vi "LS Data Loop.vi"(11 "FPGA Ref":T1) -> ()   [LabVIEW 2013]
uses:
  Controls/FPGA_Reference.ctl
  <vilib>/rvi/interface/common/niFpgaWaitOnOcc.vi
  <vilib>/Utility/error.llb/Error Cluster From Error Code.vi
  <vilib>/rvi/errors/niLvFpgaAdjustHostInterfaceError.vi
  <vilib>/rvi/interface/nirviMethod/nirviMethod.xnode
  FPGA Bitfiles/LSDurability_Main.lvbitx
  <vilib>/rvi/interface/nirviReadWriteControl/nirviReadWriteControl.xnode
  <vilib>/FPGAPlugInAG/sbRIO-9626/niLvFpga_ReadFifo_sbRIO-9626.vi
  <vilib>/rvi/errors/niLvFpgaMergeErrorWithErrorCode.vi
  NiFpgaLv.dll
panel:
  in  "LoopWait(ms) 2":u32=100
  in  "Sections 2":i32=100
  out "FIFO loops 2":i32
  out "FIFO loops":i32
  in  "LoopWait(ms)":u32=100
  in  "Sections":i32=100
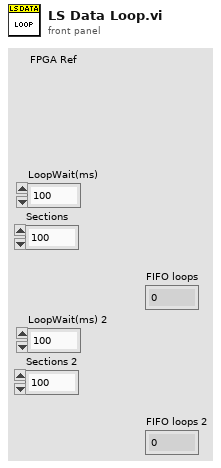
[diagram p1: front panel]
types:
  T1 = typedef "FPGA_Reference.ctl" = refnum<k20>
  T2 = cluster{"FPGA Ref":T1, "Time":dbl, "PtsTaken":i32, "Pts/File":i32, "10AveWait":u32, "Stored Filepath":path, "FileIndex":i32, "FilesUsed":i32, "Day":i32, "Anomaly Path":path}
  T3 = enum16{"open", "replace", "create", "open or create", "replace or create", "replace or create with confirmation"}
  T4 = cluster{"Running?":bool, "Profile Record":bool, "RecordInterval":i32, "RecordDuration":i32, "RecordFreq":i32, "Data Filepath":path, "Hr Record":bool, "Serial Numbers":string[]}
  T5 = typedef "LVDateTimeRec.ctl" = cluster{"fractional second":dbl, "second":i32, "minute":i32, "hour":i32, "day of month":i32, "month":i32, "year":i32, "day of week":i32, "day of year":i32, "DST":i32}
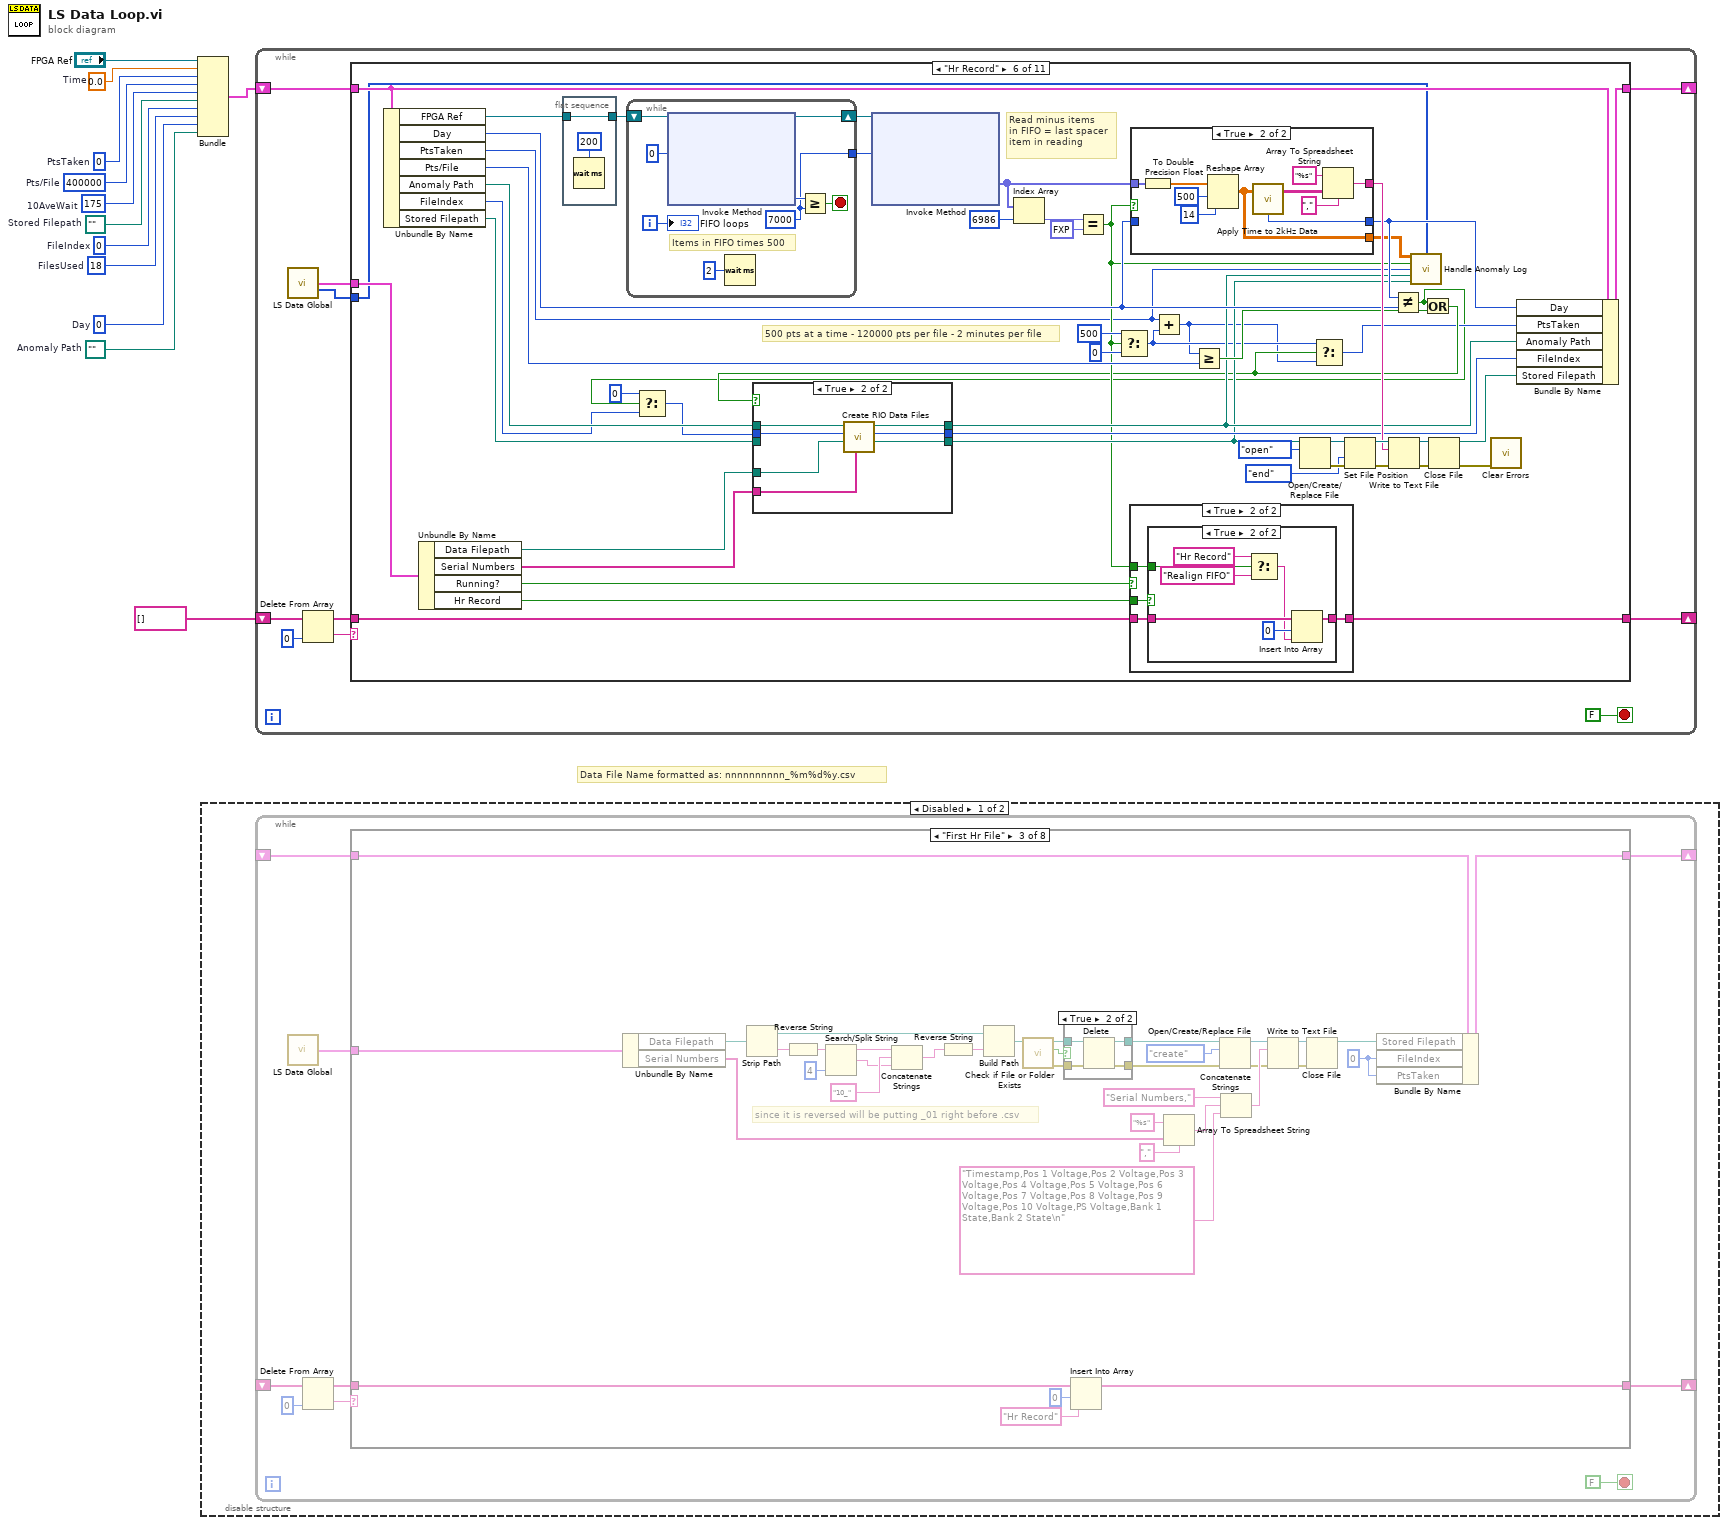
[diagram p0: block diagram]
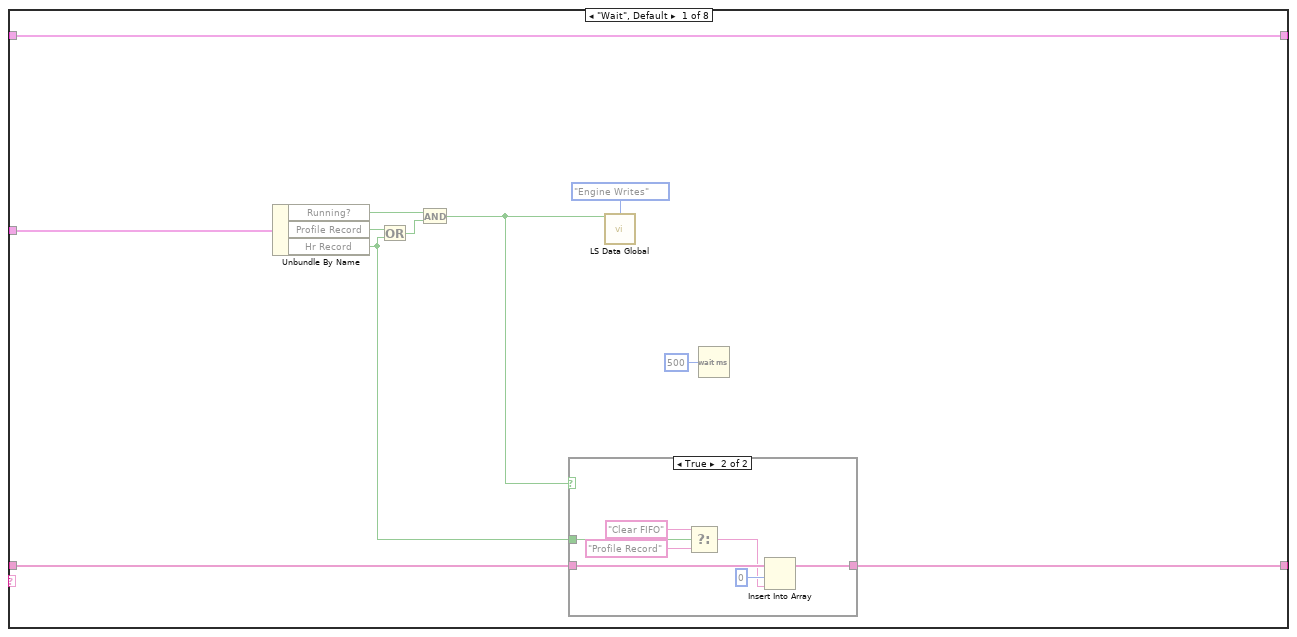
[diagram p2: hidden frame]
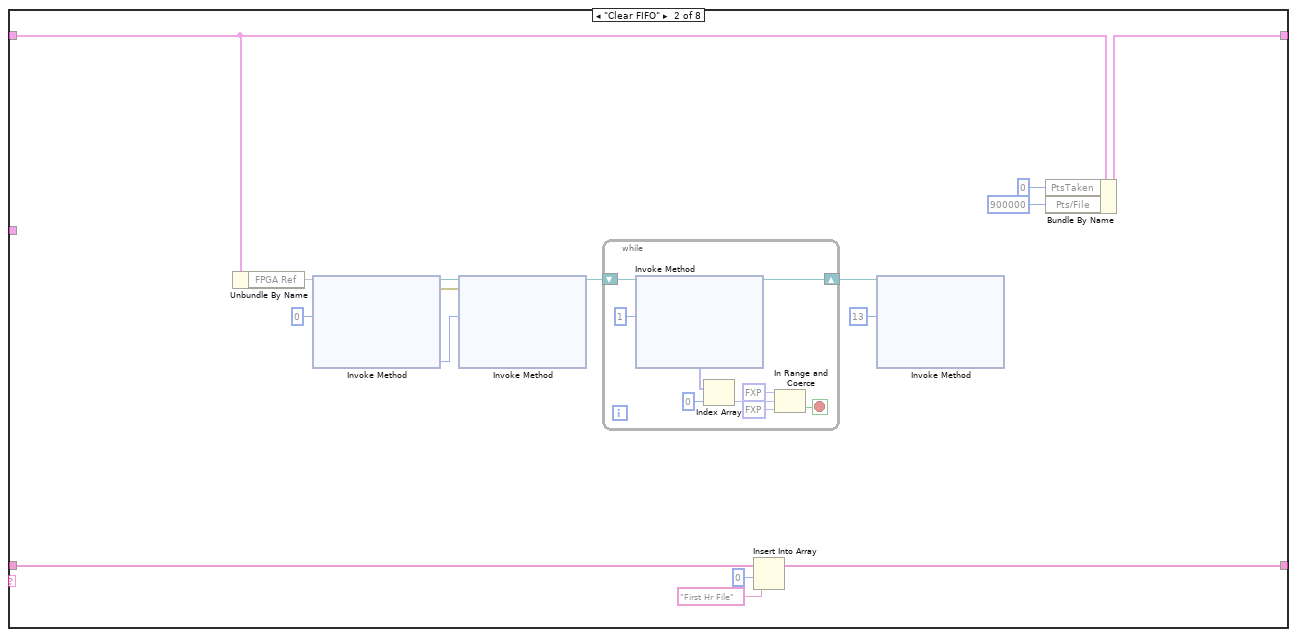
[diagram p4: hidden frame]
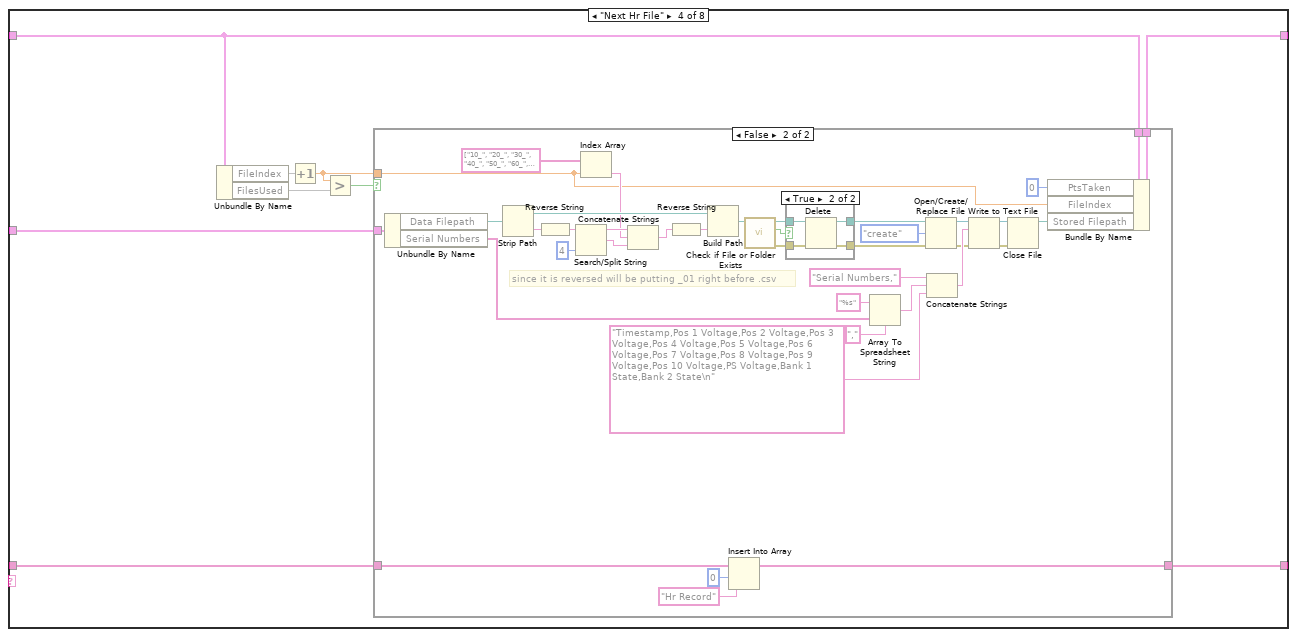
[diagram p6: hidden frame]
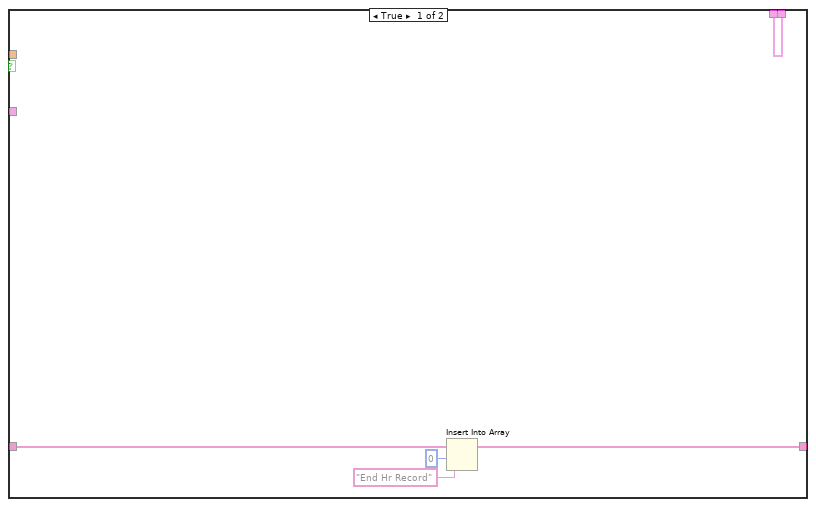
[diagram p7: hidden frame]
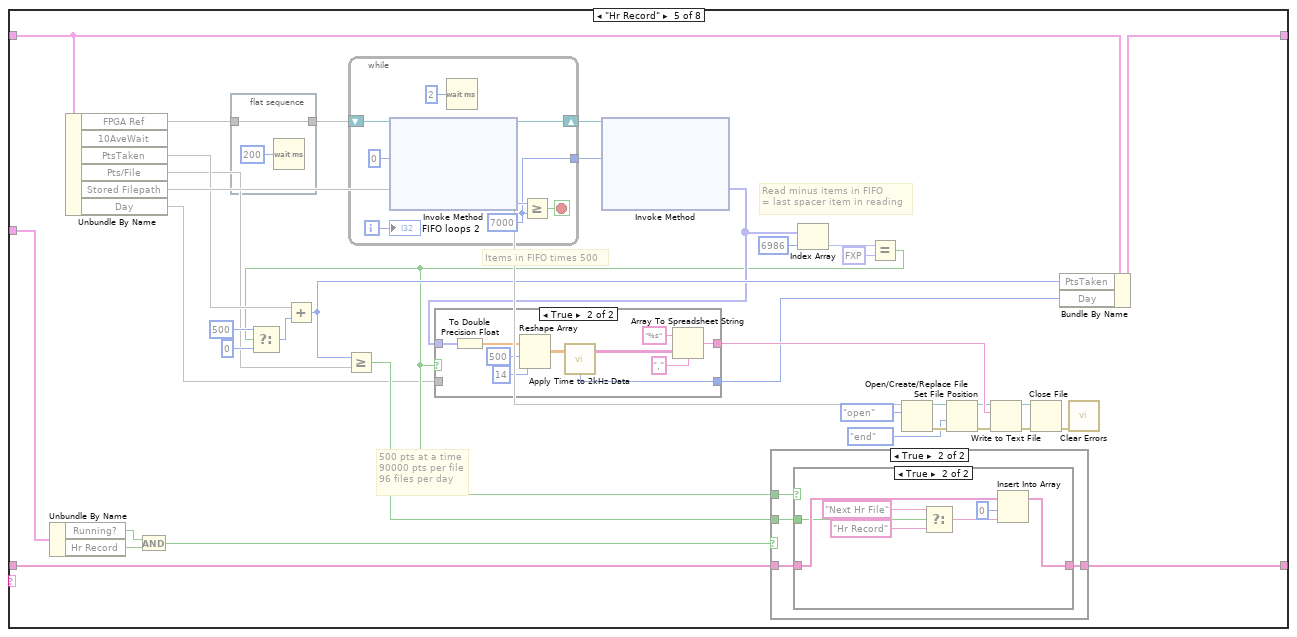
[diagram p9: hidden frame]
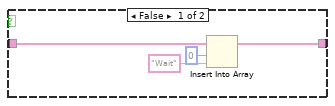
[diagram p10: hidden frame]
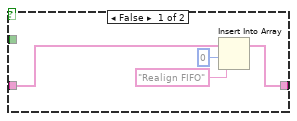
[diagram p11: hidden frame]
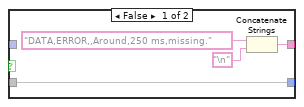
[diagram p12: hidden frame]
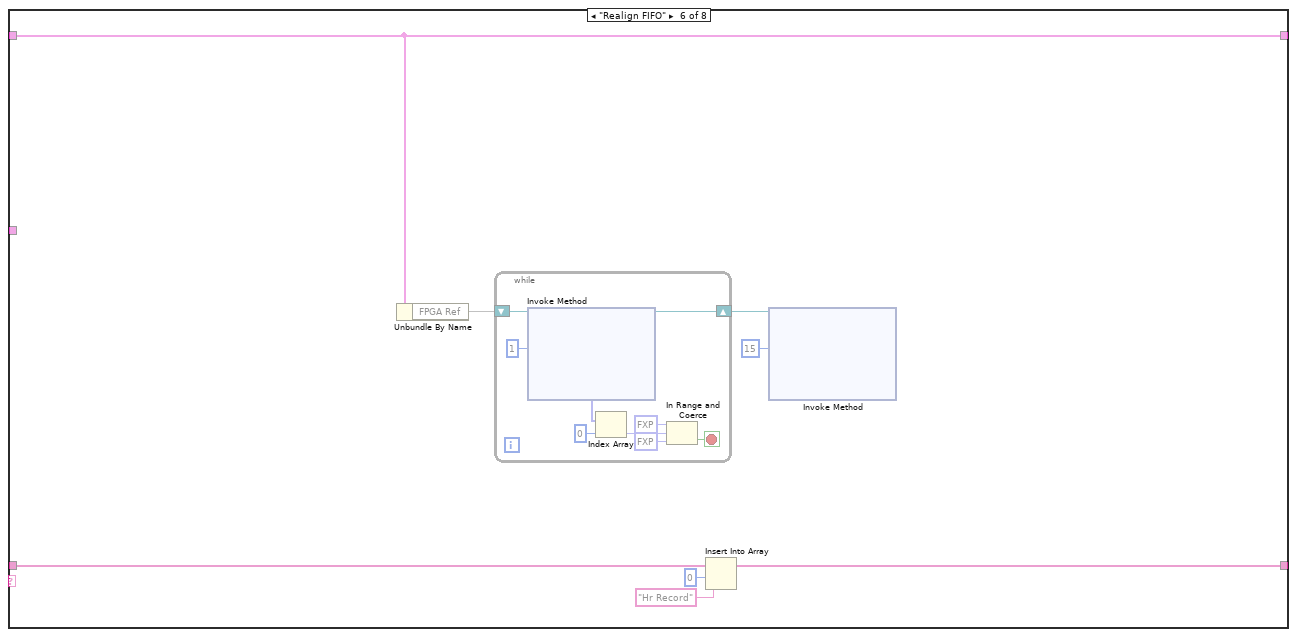
[diagram p13: hidden frame]
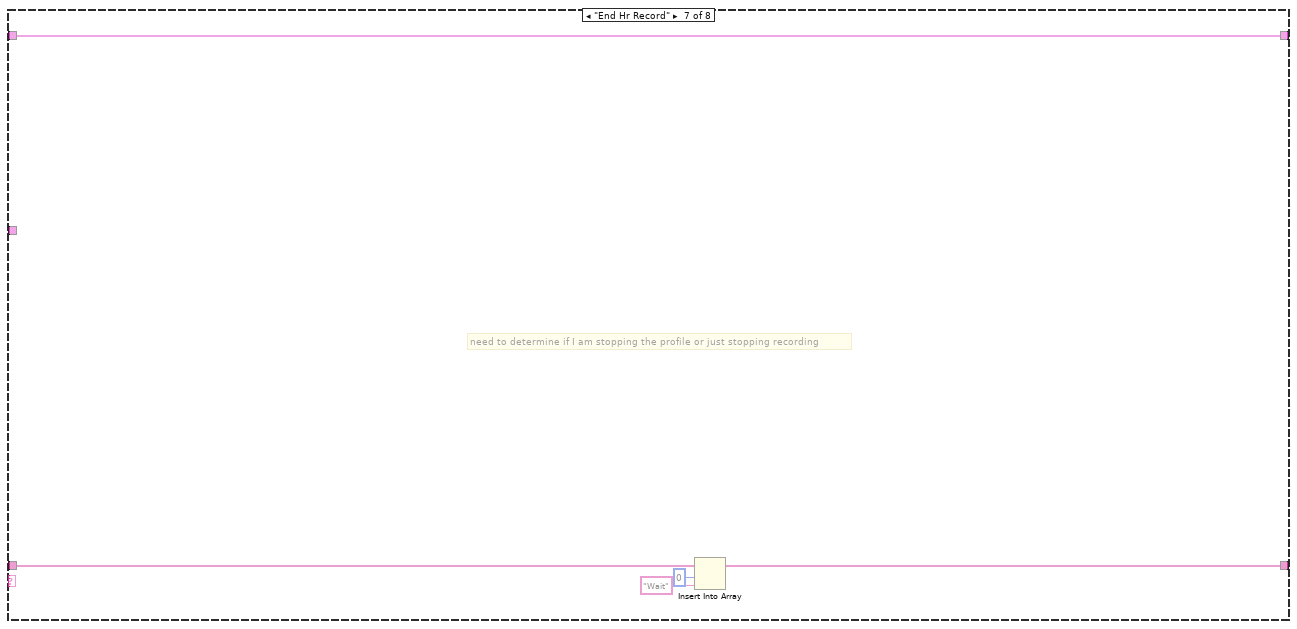
[diagram p14: hidden frame]
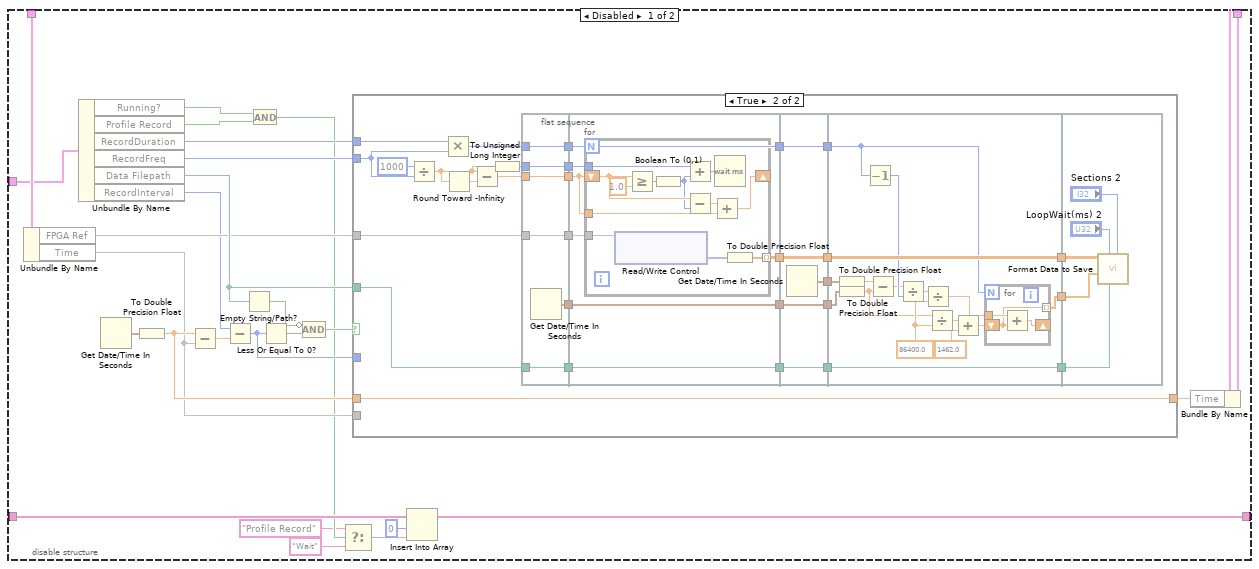
[diagram p16: hidden frame]
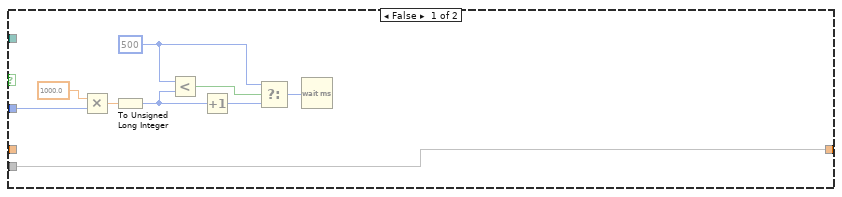
[diagram p17: hidden frame]
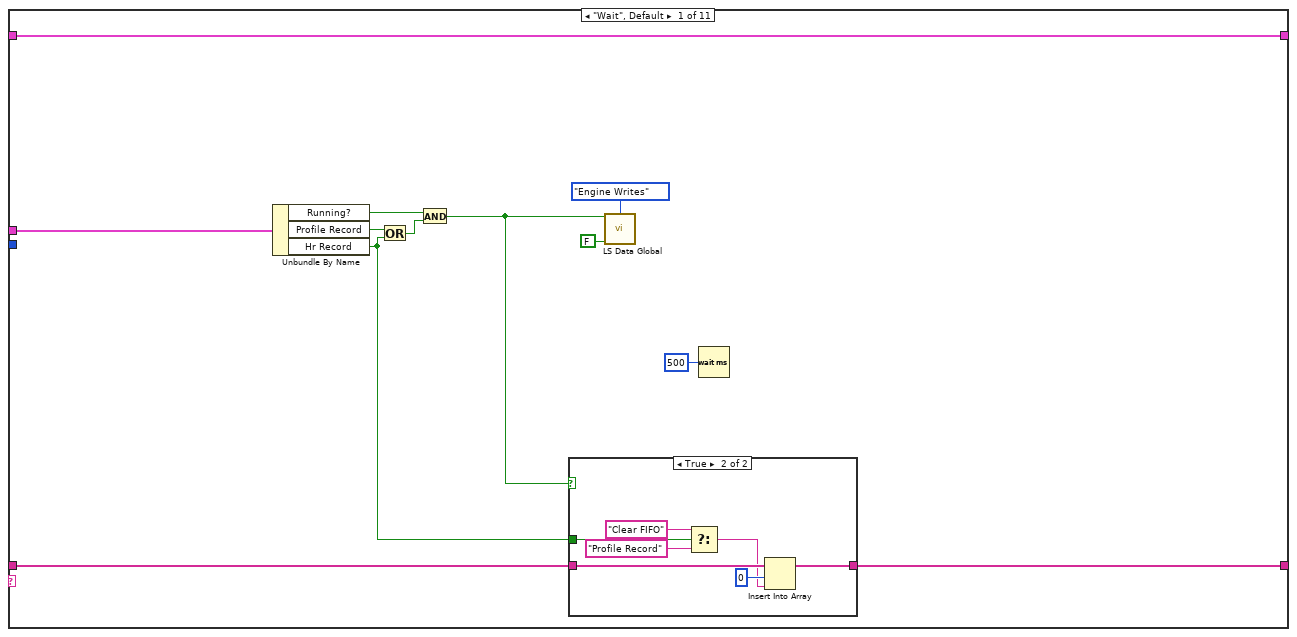
[diagram p19: hidden frame]
diagram:
  w1 = path ""  # Anomaly Path
  w2 = 0  # Day
  w3 = 18  # FilesUsed
  w4 = 0  # FileIndex
  w5 = path ""  # Stored Filepath
  w6 = u32 175  # 10AveWait
  w7 = 400000  # Pts/File
  w8 = 0  # PtsTaken
  w11 = 0.0  # Time
  # "Data File Name formatted as: nnnnnnnnnn_%m%d%y.csv"
  n1 = Bundle("FPGA Ref"="FPGA Ref", "Time"=w11, "PtsTaken"=w8, "Pts/File"=w7, "10AveWait"=w6, "Stored Filepath"=w5, "FileIndex"=w4, "FilesUsed"=w3, "Day"=w2, "Anomaly Path"=w1) -> (w10:T2)  [unwired: 1 in]
  n2 = disable-structure shown="Disabled" {
    frame Disabled {
      n3 = while {
        shift-right: [w19] -> _
        shift-left: _ -> [w20]
        shift-right: [w16] -> _
        shift-left: _ -> [w18]
        stop <- FALSE stop-if-true
        n4 = call "LS Data Global.vi"() -> ("LS Cluster Out"=w17:T4)  [unwired: 12 in, 3 out]
        n5 = Delete From Array(array=w18, index=0) -> (deleted portion=w14:string, array with subset deleted=w13:string[])  [unwired: 1 in]
        n6 = case shown="\"First Hr File\"" w14 {
          tunnel: w13 -> [w29 w51 w89 w109 w183 w249 w268 w271]
          tunnel: [w28 w49 w88 w115 w184 w248 w267 w270] -> w16
          tunnel: w17 -> [w30 _ w101 w117 w202 _ _ w272]
          tunnel: w20 -> [w27 w47 w102 w114 w178 w252 w269 w274]
          tunnel: [w27 w46 w100 w116 w177 w252 w269 w273] -> w19
          frame "Wait", Default {
            n7 = Unbundle By Name(w30) -> ("Running?"=w31:bool, "Profile Record"=w26:bool, "Hr Record"=w24:bool)
            n8 = Or(x=w26, y=w24) -> (x .or. y?=w25:bool)
            n9 = And(x=w31, y=w25) -> (x .and. y?=w22:bool)
            n10 = case shown="True" w22 {
              tunnel: w29 -> [w33 w40]
              tunnel: [w33 w39] -> w28
              tunnel: w24 -> [_ w37]
              frame False {
              }
              frame True {
                n11 = Select(t="Clear FIFO" ("new element/subarray"), s=w37, f="Profile Record" ("new element/subarray")) -> (s? t:f=w35:string)
                n12 = Insert Into Array(array=w40, index=0, new element=w35) -> (w39:string[])
              }
            }
            n13 = call "LS Data Global.vi"("Recording In"=w22, "Mode"=enum16{"Read", "Engine Writes", "Main Writes"}."Engine Writes") -> ()  [unwired: 10 in, 4 out]
            n14 = Wait (ms)(milliseconds to wait=u32 500) -> ()  [unwired: 1 out]
          }
          frame "Clear FIFO" {
            n15 = Unbundle By Name(w47) -> ("FPGA Ref"=w56)
            n16 = xnode "Invoke Method"("FPGA VI Reference In"=w56, "Number of Elements"=u32 0) -> ("FPGA VI Reference Out"=w55:refnum<k20>, "error out"=w54:errorcluster, "Elements Remaining"=w52:u32)  [unwired: 2 in, 1 out]
            n17 = xnode "Invoke Method"("FPGA VI Reference In"=w55, "error in"=w54, "Number of Elements"=w52) -> ("FPGA VI Reference Out"=w43:refnum<k20>)  [unwired: 1 in, 3 out]
            n18 = while {
              shift-right: [w64] -> w41
              shift-left: w43 -> [w65]
              stop <- w57 stop-if-true
              n19 = xnode "Invoke Method"("FPGA VI Reference In"=w65, "Number of Elements"=u32 1) -> ("FPGA VI Reference Out"=w64:refnum<k20>, "Data"=w62:fxp<+/-,18,11>[])  [unwired: 2 in, 2 out]
              n20 = Index Array(array=w62, index=0) -> (element=w60:fxp<+/-,18,11>)
              n21 = In Range and Coerce(upper limit=fxp<+/-,18,5> -14.0, x=w60, lower limit=fxp<+/-,18,5> -15.0) -> (In Range?=w57:bool)  [unwired: 1 out]
            }
            n22 = Insert Into Array(array=w51, index=0, new element="First Hr File" ("new element/subarray")) -> (w49:string[])
            n23 = xnode "Invoke Method"("FPGA VI Reference In"=w41, "Number of Elements"=u32 13) -> ()  [unwired: 2 in, 4 out]
            n24 = Bundle By Name(cluster=w47, "PtsTaken"=0, "Pts/File"=900000 ("PtsNeeded")) -> (w46:cluster{})
          }
          frame "First Hr File" {
            w66 = 0 ("FileIndex")
            # "since it is reversed will be putting _01 right before .csv"
            n25 = Unbundle By Name(w101) -> ("Data Filepath"=w99:path, "Serial Numbers"=w67:string[])
            n26 = Strip Path(path=w99) -> (stripped path=w98:path, name=w97:string)
            n27 = Reverse String(1:w97) -> (0:w95:string)
            n28 = Search/Split String(string=w95, offset (0)=4) -> (substring before match=w93:string, match + rest of string=w90:string)  [unwired: 1 in, 1 out]
            n29 = Concatenate Strings(w93, "10_", w90) -> (w92:string)
            n30 = Reverse String(1:w92) -> (0:w96:string)
            n31 = Build Path(base path=w98, name or relative path=w96) -> (appended path=w85:path)
            n32 = call <vilib>:"Check if File or Folder Exists.vi"("path"=w85) -> ("error out"=w70:errorcluster, "file or folder exists?"=w84:bool, "dup path"=w83:path)  [unwired: 8 in]
            n33 = case shown="True" w84 {
              tunnel: w83 -> [w104 w108]
              tunnel: [w104 w107] -> w72
              tunnel: w70 -> [w103 w106]
              tunnel: [w103 w105] -> w69
              frame False {
              }
              frame True {
                n34 = Delete(path (use dialog)=w108, error in=w106) -> (deleted path=w107:path, error out=w105:errorcluster)  [unwired: 3 in, 1 out]
              }
            }
            n35 = Insert Into Array(array=w89, index=0, new element="Hr Record" ("new element/subarray")) -> (w88:string[])
            n36 = Array To Spreadsheet String(delimiter (Tab)=",", array=w67, 3:"%s" ("format string")) -> (spreadsheet string=w82:string)
            n37 = Open/Create/Replace File(file path (use dialog)=w72, error in=w69, operation (0:open)=T3."create") -> (refnum out=w76:refnum<file>, error out=w74:errorcluster)  [unwired: 3 in, 1 out]
            n38 = Concatenate Strings("Serial Numbers," ("string"), w82, "Timestamp,Pos 1 Voltage,Pos 2 Voltage,Pos 3 Voltage,Pos 4 Voltage,Pos 5 Voltage,Pos 6 Voltage,Pos 7 Voltage,Pos 8 Voltage,Pos 9 Voltage,Pos 10 Voltage,PS Voltage,Bank 1 State,Bank 2 State\n") -> (w79:string)
            n39 = Write to Text File(file (use dialog)=w76, text=w79, error in=w74) -> (refnum out=w77:refnum<file>, error out=w75:errorcluster)  [unwired: 1 in, 1 out]
            n40 = Close File(refnum=w77, error in=w75) -> (path=w71:path)  [unwired: 1 out]
            n41 = Bundle By Name(cluster=w102, "Stored Filepath"=w71, "FileIndex"=w66, "PtsTaken"=w66) -> (w100:cluster{})
          }
          frame "Next Hr File" {
            n42 = Unbundle By Name(w114) -> ("FileIndex"=w113, "FilesUsed"=w112)
            n43 = Increment(x=w113) -> (x+1=w111:dbl)
            n44 = Greater?(x=w111, y=w112) -> (0:w110:bool)
            n45 = case shown="False" w110 {
              tunnel: w117 -> [_ w161]
              tunnel: [w122 w160] -> w116
              tunnel: [w120 w149] -> w115
              tunnel: w114 -> [w122 w127]
              tunnel: w111 -> [_ w125]
              tunnel: w109 -> [w121 w150]
              frame True {
                n46 = Insert Into Array(array=w121, index=0, new element="End Hr Record" ("new element/subarray")) -> (w120:string[])
              }
              frame False {
                # "since it is reversed will be putting _01 right before .csv"
                n47 = Unbundle By Name(w161) -> ("Data Filepath"=w159:path, "Serial Numbers"=w128:string[])
                n48 = Strip Path(path=w159) -> (stripped path=w158:path, name=w157:string)
                n49 = Reverse String(1:w157) -> (0:w155:string)
                n50 = Search/Split String(string=w155, offset (0)=4) -> (substring before match=w153:string, match + rest of string=w151:string)  [unwired: 1 in, 1 out]
                n51 = Index Array(array=string[] ["10_", "20_", "30_", "40_", "50_", "60_", "70_", "80_", "90_", "01_", "11_", "21_", "31_", "41_", "51_", "61_", "71_", "81_", "91_", "02_", "12_", "22_", "32_", "42_", "52_", "62_", "72_", "82_", "92_", "03_", "13_", "23_", "33_", "43_", "53_", "63_", "73_", "83_", "93_", "04_", "14_", "24_", "34_", "44_", "54_", "64_", "74_", "84_", "94_", "05_", "15_", "25_", "35_", "45_", "55_", "65_", "75_", "85_", "95_", "06_", "16_", "26_", "36_", "46_", "56_", "66_", "76_", "86_", "96_", "07_", "17_", "27_", "37_", "47_", "57_", "67_", "77_", "87_", "97_", "08_", "18_", "28_", "38_", "48_", "58_", "68_", "78_", "88_", "98_", "09_", "19_", "29_", "39_", "49_", "59_", "69_", "79_", "89_", "99_"] ("Array 2"), index=w125) -> (element=w126:string)
                n52 = Concatenate Strings(w153, w126, w151) -> (w152:string)
                n53 = Reverse String(1:w152) -> (0:w156:string)
                n54 = Build Path(base path=w158, name or relative path=w156) -> (appended path=w146:path)
                n55 = Insert Into Array(array=w150, index=0, new element="Hr Record" ("new element/subarray")) -> (w149:string[])
                n56 = call <vilib>:"Check if File or Folder Exists.vi"("path"=w146) -> ("error out"=w131:errorcluster, "file or folder exists?"=w145:bool, "dup path"=w144:path)  [unwired: 8 in]
                n57 = case shown="True" w145 {
                  tunnel: w144 -> [w163 w167]
                  tunnel: [w163 w166] -> w133
                  tunnel: w131 -> [w162 w165]
                  tunnel: [w162 w164] -> w130
                  frame False {
                  }
                  frame True {
                    n58 = Delete(path (use dialog)=w167, error in=w165) -> (deleted path=w166:path, error out=w164:errorcluster)  [unwired: 3 in, 1 out]
                  }
                }
                n59 = Array To Spreadsheet String(delimiter (Tab)=",", array=w128, 3:"%s" ("format string")) -> (spreadsheet string=w143:string)
                n60 = Open/Create/Replace File(file path (use dialog)=w133, error in=w130, operation (0:open)=T3."create") -> (refnum out=w137:refnum<file>, error out=w135:errorcluster)  [unwired: 3 in, 1 out]
                n61 = Concatenate Strings("Serial Numbers," ("string"), w143, "Timestamp,Pos 1 Voltage,Pos 2 Voltage,Pos 3 Voltage,Pos 4 Voltage,Pos 5 Voltage,Pos 6 Voltage,Pos 7 Voltage,Pos 8 Voltage,Pos 9 Voltage,Pos 10 Voltage,PS Voltage,Bank 1 State,Bank 2 State\n") -> (w140:string)
                n62 = Write to Text File(file (use dialog)=w137, text=w140, error in=w135) -> (refnum out=w138:refnum<file>, error out=w136:errorcluster)  [unwired: 1 in, 1 out]
                n63 = Close File(refnum=w138, error in=w136) -> (path=w132:path)  [unwired: 1 out]
                n64 = Bundle By Name(cluster=w127, "PtsTaken"=0, "FileIndex"=w125, "Stored Filepath"=w132) -> (w160:cluster{})
              }
            }
          }
          frame "Hr Record" {
            # "Read minus items in FIFO\n= last spacer item in reading"
            # "Items in FIFO times 500"
            # "500 pts at a time\n90000 pts per file\n96 files per day"
            n65 = Unbundle By Name(w202) -> ("Running?"=w203:bool, "Hr Record"=w204:bool)
            n66 = Unbundle By Name(w178) -> ("FPGA Ref"=w189, "PtsTaken"=w182, "Pts/File"=w175, "Stored Filepath"=w187, "Day"=w168)  [unwired: 1 out]
            n67 = And(x=w203, y=w204) -> (x .and. y?=w185:bool)
            n68 = flat-sequence {
              tunnel: w189 -> [w239]
              tunnel: [w239] -> w188
              frame #0 {
                n69 = Wait (ms)(milliseconds to wait=u32 200) -> ()  [unwired: 1 out]
              }
            }
            n70 = while {
              tunnel: [w245] -> w201
              shift-right: [w242] -> w200
              shift-left: w188 -> [w243]
              i -> [w240]
              stop <- w244 stop-if-true
              w245 = u32 7000 ("y")
              n71 = xnode "Invoke Method"("FPGA VI Reference In"=w243, "Number of Elements"=u32 0) -> ("FPGA VI Reference Out"=w242:refnum<k20>, "Elements Remaining"=w246:u32)  [unwired: 2 in, 2 out]
              n72 = Wait (ms)(milliseconds to wait=u32 2) -> ()  [unwired: 1 out]
              n73 = Greater Or Equal?(x=w246, y=w245) -> (x >= y?=w244:bool)
              "FIFO loops 2" <- w240
            }
            n74 = xnode "Invoke Method"("FPGA VI Reference In"=w200, "Number of Elements"=w201) -> ("Data"=w173:fxp<+/-,18,11>[])  [unwired: 2 in, 3 out]
            n75 = Index Array(array=w173, index=6986) -> (element=w172:fxp<+/-,18,11>)
            n76 = Equal?(x=w172, y=fxp<+/-,18,5> -15.0) -> (x = y?=w170:bool)
            n77 = Select(t=500 ("PtsTaken"), s=w170, f=0 ("PtsTaken")) -> (s? t:f=w179:i32)
            n78 = Add(x=w182, y=w179) -> (x+y=w176:i32)
            n79 = Greater Or Equal?(x=w176, y=w175) -> (x >= y?=w174:bool)
            n80 = case shown="True" w170 {
              tunnel: [w225 w232] -> w192
              tunnel: w173 -> [_ w231]
              tunnel: [w224 w228] -> w169
              tunnel: w168 -> [w224 _]
              frame False {
                n81 = Concatenate Strings("DATA,ERROR,,Around,250 ms,missing." ("string"), "\n") -> (w225:string)
              }
              frame True {
                n82 = To Double Precision Float(number=w231) -> (double precision float=w235:dbl[])
                n83 = Reshape Array(w235, 500 ("dimension size"), 14 ("dimension size")) -> (w230:dbl[][])
                n84 = call "Apply Time to 2kHz Data.vi"("Data In"=w230) -> ("Day"=w228:i32, "Data Out"=w229:string[][])  [unwired: 2 in]
                n85 = Array To Spreadsheet String(delimiter (Tab)=",", array=w229, 3:"%s" ("format string")) -> (spreadsheet string=w232:string)
              }
            }
            n86 = case shown="True" w185 {
              tunnel: w183 -> [w207 w211]
              tunnel: [w206 w210] -> w184
              tunnel: w170 -> [_ w212]
              tunnel: w174 -> [_ w209]
              frame False {
                n87 = Insert Into Array(array=w207, index=0, new element="Wait") -> (w206:string[])
              }
              frame True {
                n88 = case shown="True" w212 {
                  tunnel: w211 -> [w216 w223]
                  tunnel: [w215 w222] -> w210
                  tunnel: w209 -> [_ w220]
                  frame False {
                    n89 = Insert Into Array(array=w216, index=0, new element="Realign FIFO" ("new element/subarray")) -> (w215:string[])
                  }
                  frame True {
                    n90 = Select(t="Next Hr File", s=w220, f="Hr Record") -> (s? t:f=w219:string)
                    n91 = Insert Into Array(array=w223, index=0, new element=w219) -> (w222:string[])
                  }
                }
              }
            }
            n92 = Open/Create/Replace File(file path (use dialog)=w187, operation (0:open)=T3."open") -> (refnum out=w195:refnum<file>, error out=w194:errorcluster)  [unwired: 4 in, 1 out]
            n93 = Set File Position(refnum=w195, from (0:start)=enum16{"start", "end", "current"}."end", error in=w194) -> (refnum out=w191:refnum<file>, error out=w190:errorcluster)  [unwired: 1 in]
            n94 = Write to Text File(file (use dialog)=w191, text=w192, error in=w190) -> (refnum out=w198:refnum<file>, error out=w199:errorcluster)  [unwired: 1 in, 1 out]
            n95 = Close File(refnum=w198, error in=w199) -> (error out=w197:errorcluster)  [unwired: 1 out]
            n96 = Bundle By Name(cluster=w178, "PtsTaken"=w176, "Day"=w169) -> (w177:cluster{})
            n97 = call <vilib>:"Clear Errors.vi"("error in (no error)"=w197) -> ()  [unwired: 6 in, 1 out]
          }
          frame "Realign FIFO" {
            n98 = Unbundle By Name(w252) -> ("FPGA Ref"=w255)
            n99 = while {
              shift-right: [w263] -> w253
              shift-left: w255 -> [w264]
              stop <- w256 stop-if-true
              n100 = xnode "Invoke Method"("FPGA VI Reference In"=w264, "Number of Elements"=u32 1) -> ("FPGA VI Reference Out"=w263:refnum<k20>, "Data"=w261:fxp<+/-,18,11>[])  [unwired: 2 in, 2 out]
              n101 = Index Array(array=w261, index=0) -> (element=w259:fxp<+/-,18,11>)
              n102 = In Range and Coerce(upper limit=fxp<+/-,18,5> -14.0, x=w259, lower limit=fxp<+/-,18,5> -15.0) -> (In Range?=w256:bool)  [unwired: 1 out]
            }
            n103 = Insert Into Array(array=w249, index=0, new element="Hr Record" ("new element/subarray")) -> (w248:string[])
            n104 = xnode "Invoke Method"("FPGA VI Reference In"=w253, "Number of Elements"=u32 15) -> ()  [unwired: 2 in, 4 out]
          }
          frame "End Hr Record" {
            # "need to determine if I am stopping the profile or just stopping recording"
            n105 = Insert Into Array(array=w268, index=0, new element="Wait" ("new element/subarray")) -> (w267:string[])
          }
          frame "Profile Record" {
            n106 = disable-structure shown="Enabled" {
              disable-tunnel: w274 -> [w300 w394]
              disable-tunnel: [w299 w394] -> w273
              disable-tunnel: w272 -> [w298 _]
              disable-tunnel: w271 -> [w281 w393]
              disable-tunnel: [w280 w393] -> w270
              frame Disabled {
                n107 = Unbundle By Name(w300) -> ("FPGA Ref"=w292, "Time"=w286)
                n108 = Unbundle By Name(w298) -> ("Running?"=w283:bool, "Profile Record"=w282:bool, "RecordDuration"=w295:i32, "RecordFreq"=w296:i32, "Data Filepath"=w297:path, "RecordInterval"=w284:i32)
                n109 = Get Date/Time In Seconds() -> (seconds since 1Jan1904=w294:timestamp)
                n110 = To Double Precision Float(number=w294) -> (double precision float=w287:dbl)
                n111 = Subtract(x=w287, y=w286) -> (x-y=w291:dbl)
                n112 = Subtract(x=w284, y=w291) -> (x-y=w285:i32)
                n113 = Empty String/Path?(string/path=w297) -> (empty?=w289:bool)
                n114 = And(x=w283, y=w282) -> (x .and. y?=w278:bool)
                n115 = Less Or Equal To 0?(x=w285) -> (x <= 0?=w290:bool)
                n116 = Compound Arithmetic op=AND(invert w289, w290) -> (w288:bool)
                n117 = Select(t="Profile Record", s=w278, f="Wait") -> (s? t:f=w275:string)
                n118 = case shown="True" w288 {
                  tunnel: w296 -> [_ w331]
                  tunnel: w295 -> [_ w337]
                  tunnel: w292 -> [_ w334]
                  tunnel: w287 -> [_ w333]
                  tunnel: [w309 w333] -> w293
                  tunnel: w286 -> [w309 _]
                  tunnel: w285 -> [w303 _]
                  tunnel: w297 -> [_ w310]
                  frame False {
                    w308 = u32 500 ("milliseconds to wait")
                    n119 = Multiply(x=1000.0 ("y"), y=w303) -> (x*y=w305:dbl)
                    n120 = To Unsigned Long Integer(number=w305) -> (unsigned 32bit integer=w302:u32)
                    n121 = Less?(x=w308, y=w302) -> (x < y?=w306:bool)
                    n122 = Increment(x=w302) -> (x+1=w301:u32)
                    n123 = Select(t=w308, s=w306, f=w301) -> (s? t:f=w307:u32)
                    n124 = Wait (ms)(milliseconds to wait=w307) -> ()  [unwired: 1 out]
                  }
                  frame True {
                    n125 = Divide(x=1000, y=w331) -> (x/y=w336:dbl)
                    n126 = Multiply(x=w337, y=w331) -> (x*y=w324:i32)
                    n127 = Round Toward -Infinity(1:w336) -> (0:w338:dbl)
                    n128 = Subtract(x=w336, y=w338) -> (x-y=w330:dbl)
                    n129 = To Unsigned Long Integer(number=w336) -> (unsigned 32bit integer=w335:u32)
                    n130 = flat-sequence {
                      tunnel: w330 -> [w341]
                      tunnel: w334 -> [w342]
                      tunnel: w335 -> [w343]
                      tunnel: w324 -> [w344]
                      tunnel: [w344] -> w329
                      tunnel: [w343] -> w328
                      tunnel: [w342] -> w327
                      tunnel: [w341] -> w326
                      tunnel: [w340] -> w319
                      tunnel: [w339] -> w311
                      tunnel: w310 -> [w339]
                      tunnel: w329 -> [w347]
                      tunnel: w328 -> [w351]
                      tunnel: w327 -> [w350]
                      tunnel: w326 -> [w345]
                      tunnel: [w349] -> w325
                      tunnel: [w348] -> w320
                      tunnel: w319 -> [w348]
                      tunnel: [w347] -> w317
                      tunnel: [w346] -> w312
                      tunnel: w311 -> [w346]
                      tunnel: w325 -> [w368]
                      tunnel: [w368] -> w323
                      tunnel: [w367] -> w322
                      tunnel: [w366] -> w321
                      tunnel: w320 -> [w366]
                      tunnel: [w365] -> w318
                      tunnel: w317 -> [w365]
                      tunnel: [w364] -> w313
                      tunnel: w312 -> [w364]
                      tunnel: w323 -> [w384]
                      tunnel: w322 -> [w378]
                      tunnel: w321 -> [w377]
                      tunnel: w318 -> [w376]
                      tunnel: [w384] -> w316
                      tunnel: [w374] -> w315
                      tunnel: [w371] -> w314
                      tunnel: w313 -> [w371]
                      tunnel: w314 -> [w390]
                      tunnel: w315 -> [w391]
                      tunnel: w316 -> [w392]
                      frame #0 {
                        n131 = Get Date/Time In Seconds() -> (seconds since 1Jan1904=w340:timestamp)
                      }
                      frame #1 {
                        n132 = for {
                          N: w347 -> [_]
                          tunnel: w351 -> [w363]
                          shift-right: [w360] -> _
                          shift-left: w345 -> [w361]
                          tunnel: w345 -> [w359]
                          tunnel: w350 -> [w358]
                          tunnel: [w356] -> w349 mode=indexing
                          n133 = xnode "Read/Write Control"("FPGA VI Reference In"=w358) -> ("Analog Inputs"=w357:fxp<+/-,28,17>[])  [unwired: 1 in, 2 out]
                          n134 = Greater Or Equal?(x=w361, y=1.0) -> (x >= y?=w354:bool)
                          n135 = Boolean To (0,1)(Boolean=w354) -> (0, 1=w353:i16)
                          n136 = Add(x=w363, y=w353) -> (x+y=w362:u32)
                          n137 = Subtract(x=w361, y=w353) -> (x-y=w352:dbl)
                          n138 = Add(x=w352, y=w359) -> (x+y=w360:dbl)
                          n139 = Wait (ms)(milliseconds to wait=w362) -> ()  [unwired: 1 out]
                          n140 = To Double Precision Float(number=w357) -> (double precision float=w356:dbl[])
                        }
                      }
                      frame #2 {
                        n141 = Get Date/Time In Seconds() -> (seconds since 1Jan1904=w367:timestamp)
                      }
                      frame #3 {
                        w373 = 86400.0 ("y")
                        n142 = To Double Precision Float(number=w378) -> (double precision float=w372:dbl)
                        n143 = To Double Precision Float(number=w377) -> (double precision float=w369:dbl)
                        n144 = Decrement(x=w376) -> (x-1=w375:i32)
                        n145 = Subtract(x=w372, y=w369) -> (x-y=w370:dbl)
                        n146 = Divide(x=w370, y=w375) -> (x/y=w379:dbl)
                        n147 = Divide(x=w379, y=w373) -> (x/y=w383:dbl)
                        n148 = Divide(x=w369, y=w373) -> (x/y=w380:dbl)
                        n149 = Add(x=w380, y=1462.0) -> (x+y=w382:dbl)
                        n150 = for {
                          N: w376 -> [_]
                          shift-right: [w385] -> _
                          shift-left: w382 -> [w386]
                          tunnel: w383 -> [w387]
                          tunnel: [w386] -> w374 mode=indexing
                          n151 = Add(x=w387, y=w386) -> (x+y=w385:dbl)
                        }
                      }
                      frame #4 {
                        n152 = call "Format Data to Save.vi"("Sections"="Sections 2", "FilePath"=w390, "LoopBeginWait(ms)"="LoopWait(ms) 2", "Time"=w391, "Data"=w392) -> ()  [unwired: 7 in]
                      }
                    }
                  }
                }
                n153 = Insert Into Array(array=w281, index=0, new element=w275) -> (w280:string[])
                n154 = Bundle By Name(cluster=w300, "Time"=w293) -> (w299:cluster{})
              }
              frame Enabled {
              }
            }
          }
        }
      }
    }
    frame Enabled {
    }
  }
  n155 = while {
    shift-right: [w402] -> _
    shift-left: w10 -> [w403]
    shift-right: [w399] -> _
    shift-left: string[] [] -> [w401]
    stop <- FALSE stop-if-true
    n156 = call "LS Data Global.vi"() -> ("LS Cluster Out"=w400:T4, "Anomalies Out"=w395:i32[])  [unwired: 12 in, 2 out]
    n157 = Delete From Array(array=w401, index=0) -> (deleted portion=w397:string, array with subset deleted=w396:string[])  [unwired: 1 in]
    n158 = case shown="\"Hr Record\"" w397 {
      tunnel: w396 -> [w413 w433 w458 w516 w573 w644 w742 w745 w769 w778 w781]
      tunnel: [w412 w432 w456 w515 w579 w643 w742 w744 w768 w777 w780] -> w399
      tunnel: w400 -> [w414 w434 _ w518 w581 w682 _ _ _ _ w782]
      tunnel: w403 -> [w411 w431 w454 w512 w578 w665 w743 w748 w765 w779 w784]
      tunnel: [w411 w431 w453 w517 w580 w664 w743 w748 w765 w779 w783] -> w402
      tunnel: w395 -> [_ _ _ _ _ w632 _ _ _ _ _]
      frame "Wait", Default {
        n159 = Unbundle By Name(w414) -> ("Running?"=w415:bool, "Profile Record"=w410:bool, "Hr Record"=w408:bool)
        n160 = Or(x=w410, y=w408) -> (x .or. y?=w409:bool)
        n161 = And(x=w415, y=w409) -> (x .and. y?=w406:bool)
        n162 = case shown="True" w406 {
          tunnel: w413 -> [w417 w424]
          tunnel: [w417 w423] -> w412
          tunnel: w408 -> [_ w421]
          frame False {
          }
          frame True {
            n163 = Select(t="Clear FIFO" ("new element/subarray"), s=w421, f="Profile Record" ("new element/subarray")) -> (s? t:f=w419:string)
            n164 = Insert Into Array(array=w424, index=0, new element=w419) -> (w423:string[])
          }
        }
        n165 = call "LS Data Global.vi"("Recording In"=w406, "Mode"=enum16{"Read", "Engine Writes", "Main Writes"}."Engine Writes", "Transferring In"=FALSE) -> ()  [unwired: 9 in, 4 out]
        n166 = Wait (ms)(milliseconds to wait=u32 500) -> ()  [unwired: 1 out]
      }
      frame "Wait 2" {
        # "This wait is used to keep the files going from one cycle to the next when recording is based on profile"
        n167 = Unbundle By Name(w434) -> ("Running?"=w435:bool, "Profile Record"=w430:bool, "Hr Record"=w428:bool)
        n168 = Or(x=w430, y=w428) -> (x .or. y?=w429:bool)
        n169 = And(x=w435, y=w429) -> (x .and. y?=w426:bool)
        n170 = case shown="True" w426 {
          tunnel: w433 -> [w440 w447]
          tunnel: [w439 w446] -> w432
          tunnel: w428 -> [_ w444]
          frame False {
            n171 = Insert Into Array(array=w440, index=0, new element="Wait 2" ("new element/subarray")) -> (w439:string[])
          }
          frame True {
            n172 = Select(t=string[] ["Empty FIFO", "Realign FIFO"], s=w444, f=string[] ["Profile Record"]) -> (s? t:f=w443:string[])
            n173 = Insert Into Array(array=w447, index=0, new element=w443) -> (w446:string[])
          }
        }
        n174 = call "LS Data Global.vi"("Recording In"=w426, "Mode"=enum16{"Read", "Engine Writes", "Main Writes"}."Engine Writes", "Transferring In"=FALSE) -> ()  [unwired: 9 in, 4 out]
        n175 = Wait (ms)(milliseconds to wait=u32 500) -> ()  [unwired: 1 out]
      }
      frame "Clear FIFO" {
        n176 = Unbundle By Name(w454) -> ("FPGA Ref"=w463:T1)
        n177 = xnode "Invoke Method"("FPGA VI Reference In"=w463, "Number of Elements"=u32 0) -> ("FPGA VI Reference Out"=w462:T1, "error out"=w461:errorcluster, "Elements Remaining"=w459:u32)  [unwired: 2 in, 1 out]
        n178 = xnode "Invoke Method"("FPGA VI Reference In"=w462, "error in"=w461, "Number of Elements"=w459) -> ("FPGA VI Reference Out"=w450:T1)  [unwired: 1 in, 3 out]
        n179 = while {
          shift-right: [w471] -> w448
          shift-left: w450 -> [w472]
          stop <- w464 stop-if-true
          n180 = xnode "Invoke Method"("FPGA VI Reference In"=w472, "Number of Elements"=u32 1) -> ("FPGA VI Reference Out"=w471:T1, "Data"=w469:fxp<+/-,18,11>[])  [unwired: 2 in, 2 out]
          n181 = Index Array(array=w469, index=0) -> (element=w467:fxp<+/-,18,11>)
          n182 = In Range and Coerce(upper limit=fxp<+/-,18,5> -14.0, x=w467, lower limit=fxp<+/-,18,5> -15.0) -> (In Range?=w464:bool)  [unwired: 1 out]
        }
        n183 = Insert Into Array(array=w458, index=0, new element="First Hr File" ("new element/subarray")) -> (w456:string[])
        n184 = xnode "Invoke Method"("FPGA VI Reference In"=w448, "Number of Elements"=u32 13) -> ()  [unwired: 2 in, 4 out]
        n185 = Bundle By Name(cluster=w454, "PtsTaken"=0, "Pts/File"=120000 ("PtsNeeded")) -> (w453:T2)
      }
      frame "First Hr File" {
        w474 = 0
        n186 = Unbundle By Name(w518) -> ("Data Filepath"=w497:path, "Serial Numbers"=w486:string[])
        n187 = Get Date/Time In Seconds() -> (seconds since 1Jan1904=w476:timestamp)
        n188 = Format Date/Time String(time format string (%c)="_%m%d%y", seconds (now)=w476) -> (date/time string=w482:string)  [unwired: 1 in]
        n189 = Strip Path(path=w497) -> (name=w509:string)  [unwired: 1 out]
        n190 = String Subset(string=w482, offset (0)=1) -> (substring=w507:string)  [unwired: 1 in]
        n191 = Build Path(base path=w497, name or relative path=w507) -> (appended path=w495:path)
        n192 = Concatenate Strings(w509, ".csv" ("string")) -> (w511:string)
        n193 = Seconds To Date/Time(time stamp (now)=w476) -> (date time rec=w477:T5)  [unwired: 1 in]
        n194 = call "File Indexer.vi"("File Index In"=w474) -> ("File Indicator Out"=w473:string)  [unwired: 10 in]
        n195 = Create Folder(path (use dialog)=w495) -> (created path=w478:path, error out=w496:errorcluster)  [unwired: 2 in, 1 out]
        n196 = String Length(string=w511) -> (length=w503:i32)
        n197 = Unbundle By Name(w477) -> ("day of month"=w475:i32)
        n198 = call <vilib>:"Clear Errors.vi"("error in (no error)"=w496) -> ()  [unwired: 6 in, 1 out]
        n199 = Subtract(x=w503, y=4) -> (x-y=w505:i32)
        n200 = Search/Split String(string=w511, offset (0)=w505) -> (substring before match=w483:string, match + rest of string=w479:string)  [unwired: 1 in, 1 out]
        n201 = Insert Into Array(array=w516, index=0, new element="Hr Record" ("new element/subarray")) -> (w515:string[])
        n202 = Concatenate Strings(w483, w482) -> (w480:string)
        n203 = Concatenate Strings(w483, "_Anomaly Log" ("string"), w482, w479) -> (w493:string)
        n204 = Concatenate Strings(w480, w473, w479) -> (w481:string)
        n205 = Build Path(base path=w478, name or relative path=w493) -> (appended path=w491:path)
        n206 = Increment(x=w474) -> (x+1=w485:i32)
        n207 = Build Path(base path=w478, name or relative path=w481) -> (appended path=w502:path)
        n208 = call <vilib>:"Check if File or Folder Exists.vi"("path"=w491) -> ("error out"=w488:errorcluster, "file or folder exists?"=w490:bool, "dup path"=w489:path)  [unwired: 8 in]
        n209 = call <vilib>:"Check if File or Folder Exists.vi"("path"=w502) -> ("error out"=w499:errorcluster, "file or folder exists?"=w501:bool, "dup path"=w500:path)  [unwired: 8 in]
        n210 = case shown="True" w501 {
          tunnel: w500 -> [w539 _]
          tunnel: [w538 w546] -> w494
          tunnel: w499 -> [w537 _]
          tunnel: w486 -> [w531 w553]
          tunnel: w485 -> [w529 _]
          tunnel: [w529 w559] -> w484
          tunnel: w480 -> [_ w561]
          tunnel: w479 -> [_ w560]
          tunnel: w478 -> [_ w562]
          frame False {
            n211 = Open/Create/Replace File(file path (use dialog)=w539, error in=w537, operation (0:open)=T3."create") -> (refnum out=w541:refnum<file>, error out=w543:errorcluster)  [unwired: 3 in, 1 out]
            n212 = Array To Spreadsheet String(delimiter (Tab)=",", array=w531, 3:"%s" ("format string")) -> (spreadsheet string=w532:string)
            n213 = Concatenate Strings("Serial Numbers," ("string"), w532, "Timestamp,Pos 1 Voltage,Pos 2 Voltage,Pos 3 Voltage,Pos 4 Voltage,Pos 5 Voltage,Pos 6 Voltage,Pos 7 Voltage,Pos 8 Voltage,Pos 9 Voltage,Pos 10 Voltage,PS Voltage,Bank 1 State,Bank 2 State\n") -> (w530:string)
            n214 = Write to Text File(file (use dialog)=w541, text=w530, error in=w543) -> (refnum out=w540:refnum<file>, error out=w542:errorcluster)  [unwired: 1 in, 1 out]
            n215 = Close File(refnum=w540, error in=w542) -> (path=w538:path)  [unwired: 1 out]
          }
          frame True {
            n216 = while {
              tunnel: w562 -> [w572]
              tunnel: w561 -> [w571]
              tunnel: w560 -> [w570]
              tunnel: [w567] -> w547
              tunnel: [w565] -> w559
              i -> [w566]
              stop <- w568 continue-if-true
              n217 = Increment(x=w566) -> (x+1=w564:i32)
              n218 = Increment(x=w564) -> (x+1=w565:i32)
              n219 = call "File Indexer.vi"("File Index In"=w564) -> ("File Indicator Out"=w563:string)  [unwired: 10 in]
              n220 = Concatenate Strings(w571, w563, w570) -> (w569:string)
              n221 = Build Path(base path=w572, name or relative path=w569) -> (appended path=w567:path)
              n222 = call <vilib>:"Check if File or Folder Exists.vi"("path"=w567) -> ("file or folder exists?"=w568:bool)  [unwired: 8 in, 2 out]
            }
            n223 = Array To Spreadsheet String(delimiter (Tab)=",", array=w553, 3:"%s" ("format string")) -> (spreadsheet string=w554:string)
            n224 = Concatenate Strings("Serial Numbers," ("string"), w554, "Timestamp,Pos 1 Voltage,Pos 2 Voltage,Pos 3 Voltage,Pos 4 Voltage,Pos 5 Voltage,Pos 6 Voltage,Pos 7 Voltage,Pos 8 Voltage,Pos 9 Voltage,Pos 10 Voltage,PS Voltage,Bank 1 State,Bank 2 State\n") -> (w545:string)
            n225 = Open/Create/Replace File(file path (use dialog)=w547, operation (0:open)=T3."create") -> (refnum out=w549:refnum<file>, error out=w551:errorcluster)  [unwired: 4 in, 1 out]
            n226 = Write to Text File(file (use dialog)=w549, text=w545, error in=w551) -> (refnum out=w548:refnum<file>, error out=w550:errorcluster)  [unwired: 1 in, 1 out]
            n227 = Close File(refnum=w548, error in=w550) -> (path=w546:path)  [unwired: 1 out]
          }
        }
        n228 = case shown="False" w490 {
          tunnel: w489 -> [w521 w528]
          tunnel: [w522 w528] -> w498
          tunnel: w488 -> [w520 _]
          tunnel: "LS Position,Anomaly Count,Filename,File Row Index,Voltage Delta\n" -> [w519 _]
          frame False {
            n229 = Open/Create/Replace File(file path (use dialog)=w521, error in=w520, operation (0:open)=T3."create") -> (refnum out=w524:refnum<file>, error out=w526:errorcluster)  [unwired: 3 in, 1 out]
            n230 = Write to Text File(file (use dialog)=w524, text=w519, error in=w526) -> (refnum out=w523:refnum<file>, error out=w525:errorcluster)  [unwired: 1 in, 1 out]
            n231 = Close File(refnum=w523, error in=w525) -> (path=w522:path)  [unwired: 1 out]
          }
          frame True {
          }
        }
        n232 = Bundle By Name(cluster=w512, "Anomaly Path"=w498, "FileIndex"=w484, "Stored Filepath"=w494, "Day"=w475) -> (w517:T2)
      }
      frame "Next Hr File" {
        n233 = Unbundle By Name(w578) -> ("FileIndex"=w577:i32, "FilesUsed"=w576:i32)
        n234 = Increment(x=w577) -> (x+1=w575:i32)
        n235 = Greater?(x=w575, y=w576) -> (0:w574:bool)
        n236 = case shown="False" w574 {
          tunnel: w581 -> [_ w625]
          tunnel: [w586 w624] -> w580
          tunnel: [w584 w613] -> w579
          tunnel: w578 -> [w586 w591]
          tunnel: w575 -> [_ w589]
          tunnel: w573 -> [w585 w614]
          frame True {
            n237 = Insert Into Array(array=w585, index=0, new element="End Hr Record" ("new element/subarray")) -> (w584:string[])
          }
          frame False {
            # "since it is reversed will be putting _01 right before .csv"
            n238 = Unbundle By Name(w625) -> ("Data Filepath"=w623:path, "Serial Numbers"=w592:string[])
            n239 = Strip Path(path=w623) -> (stripped path=w622:path, name=w621:string)
            n240 = Reverse String(1:w621) -> (0:w619:string)
            n241 = Search/Split String(string=w619, offset (0)=4) -> (substring before match=w617:string, match + rest of string=w615:string)  [unwired: 1 in, 1 out]
            n242 = Index Array(array=string[] ["10_", "20_", "30_", "40_", "50_", "60_", "70_", "80_", "90_", "01_", "11_", "21_", "31_", "41_", "51_", "61_", "71_", "81_", "91_", "02_", "12_", "22_", "32_", "42_", "52_", "62_", "72_", "82_", "92_", "03_", "13_", "23_", "33_", "43_", "53_", "63_", "73_", "83_", "93_", "04_", "14_", "24_", "34_", "44_", "54_", "64_", "74_", "84_", "94_", "05_", "15_", "25_", "35_", "45_", "55_", "65_", "75_", "85_", "95_", "06_", "16_", "26_", "36_", "46_", "56_", "66_", "76_", "86_", "96_", "07_", "17_", "27_", "37_", "47_", "57_", "67_", "77_", "87_", "97_", "08_", "18_", "28_", "38_", "48_", "58_", "68_", "78_", "88_", "98_", "09_", "19_", "29_", "39_", "49_", "59_", "69_", "79_", "89_", "99_"] ("Array 2"), index=w589) -> (element=w590:string)
            n243 = Concatenate Strings(w617, w590, w615) -> (w616:string)
            n244 = Reverse String(1:w616) -> (0:w620:string)
            n245 = Build Path(base path=w622, name or relative path=w620) -> (appended path=w610:path)
            n246 = Insert Into Array(array=w614, index=0, new element="Hr Record" ("new element/subarray")) -> (w613:string[])
            n247 = call <vilib>:"Check if File or Folder Exists.vi"("path"=w610) -> ("error out"=w595:errorcluster, "file or folder exists?"=w609:bool, "dup path"=w608:path)  [unwired: 8 in]
            n248 = case shown="True" w609 {
              tunnel: w608 -> [w627 w631]
              tunnel: [w627 w630] -> w597
              tunnel: w595 -> [w626 w629]
              tunnel: [w626 w628] -> w594
              frame False {
              }
              frame True {
                n249 = Delete(path (use dialog)=w631, error in=w629) -> (deleted path=w630:path, error out=w628:errorcluster)  [unwired: 3 in, 1 out]
              }
            }
            n250 = Array To Spreadsheet String(delimiter (Tab)=",", array=w592, 3:"%s" ("format string")) -> (spreadsheet string=w607:string)
            n251 = Open/Create/Replace File(file path (use dialog)=w597, error in=w594, operation (0:open)=T3."create") -> (refnum out=w601:refnum<file>, error out=w599:errorcluster)  [unwired: 3 in, 1 out]
            n252 = Concatenate Strings("Serial Numbers," ("string"), w607, "Timestamp,Pos 1 Voltage,Pos 2 Voltage,Pos 3 Voltage,Pos 4 Voltage,Pos 5 Voltage,Pos 6 Voltage,Pos 7 Voltage,Pos 8 Voltage,Pos 9 Voltage,Pos 10 Voltage,PS Voltage,Bank 1 State,Bank 2 State\n") -> (w604:string)
            n253 = Write to Text File(file (use dialog)=w601, text=w604, error in=w599) -> (refnum out=w602:refnum<file>, error out=w600:errorcluster)  [unwired: 1 in, 1 out]
            n254 = Close File(refnum=w602, error in=w600) -> (path=w596:path)  [unwired: 1 out]
            n255 = Bundle By Name(cluster=w591, "PtsTaken"=0, "FileIndex"=w589, "Stored Filepath"=w596) -> (w624:T2)
          }
        }
      }
      frame "Hr Record" {
        # "Read minus items\nin FIFO = last spacer\nitem in reading"
        # "500 pts at a time - 120000 pts per file - 2 minutes per file"
        n256 = Unbundle By Name(w665) -> ("FPGA Ref"=w670:T1, "Day"=w657:i32, "PtsTaken"=w641:i32, "Pts/File"=w663:i32, "Anomaly Path"=w655:path, "FileIndex"=w635:i32, "Stored Filepath"=w654:path)
        n257 = Unbundle By Name(w682) -> ("Data Filepath"=w642:path, "Serial Numbers"=w651:string[], "Running?"=w646:bool, "Hr Record"=w645:bool)
        n258 = flat-sequence {
          tunnel: w670 -> [w728]
          tunnel: [w728] -> w669
          frame #0 {
            n259 = Wait (ms)(milliseconds to wait=u32 200) -> ()  [unwired: 1 out]
          }
        }
        n260 = while {
          tunnel: [w734] -> w681
          shift-right: [w731] -> w680
          shift-left: w669 -> [w732]
          i -> [w730]
          stop <- w733 stop-if-true
          w734 = u32 7000 ("y")
          # "Items in FIFO times 500"
          n261 = xnode "Invoke Method"("FPGA VI Reference In"=w732, "Number of Elements"=u32 0) -> ("FPGA VI Reference Out"=w731:T1, "Elements Remaining"=w735:u32)  [unwired: 2 in, 2 out]
          n262 = Wait (ms)(milliseconds to wait=u32 2) -> ()  [unwired: 1 out]
          n263 = Greater Or Equal?(x=w735, y=w734) -> (x >= y?=w733:bool)
          "FIFO loops" <- w730
        }
        n264 = xnode "Invoke Method"("FPGA VI Reference In"=w680, "Number of Elements"=w681) -> ("Data"=w662:fxp<+/-,18,11>[])  [unwired: 2 in, 3 out]
        n265 = Index Array(array=w662, index=6986) -> (element=w661:fxp<+/-,18,11>)
        n266 = Equal?(x=w661, y=fxp<+/-,18,5> -15.0) -> (x = y?=w647:bool)
        n267 = Select(t=500 ("PtsTaken"), s=w647, f=0 ("PtsTaken")) -> (s? t:f=w639:i32)
        n268 = case shown="True" w646 {
          tunnel: w644 -> [w685 w690]
          tunnel: [w684 w689] -> w643
          tunnel: w647 -> [_ w687]
          tunnel: w645 -> [_ w688]
          frame False {
            n269 = Insert Into Array(array=w685, index=0, new element="Wait") -> (w684:string[])
          }
          frame True {
            n270 = case shown="True" w688 {
              tunnel: w690 -> [w694 w701]
              tunnel: [w693 w700] -> w689
              tunnel: w687 -> [_ w698]
              frame False {
                n271 = Insert Into Array(array=w694, index=0, new element="Transfer Files") -> (w693:string[])
              }
              frame True {
                n272 = Select(t="Hr Record", s=w698, f="Realign FIFO" ("new element/subarray")) -> (s? t:f=w696:string)
                n273 = Insert Into Array(array=w701, index=0, new element=w696) -> (w700:string[])
              }
            }
          }
        }
        n274 = case shown="True" w647 {
          tunnel: [w714 w721] -> w659
          tunnel: w662 -> [_ w720]
          tunnel: [w713 w718] -> w658
          tunnel: w657 -> [w713 _]
          tunnel: [dbl[][] [] w717] -> w650
          frame False {
            n275 = Concatenate Strings("DATA,ERROR,,Around,250 ms,missing." ("string"), "\n") -> (w714:string)
          }
          frame True {
            n276 = To Double Precision Float(number=w720) -> (double precision float=w724:dbl[])
            n277 = Reshape Array(w724, 500 ("dimension size"), 14 ("dimension size")) -> (w717:dbl[][])
            n278 = call "Apply Time to 2kHz Data.vi"("Data In"=w717) -> ("Day"=w718:i32, "Data Out"=w719:string[][])  [unwired: 2 in]
            n279 = Array To Spreadsheet String(delimiter (Tab)=",", array=w719, 3:"%s" ("format string")) -> (spreadsheet string=w721:string)
          }
        }
        n280 = Add(x=w641, y=w639) -> (x+y=w638:i32)
        n281 = Greater Or Equal?(x=w638, y=w663) -> (x >= y?=w656:bool)
        n282 = Not Equal?(x=w658, y=w657) -> (x != y?=w636:bool)
        n283 = Select(t=0, s=w636, f=w635) -> (s? t:f=w634:i32)
        n284 = Or(x=w636, y=w656) -> (x .or. y?=w640:bool)
        n285 = case shown="True" w640 {
          tunnel: w654 -> [w704 _]
          tunnel: [w704 w711] -> w648
          tunnel: w655 -> [w703 w710]
          tunnel: [w703 w709] -> w649
          tunnel: w634 -> [w702 w708]
          tunnel: [w702 w707] -> w652
          tunnel: w651 -> [_ w706]
          tunnel: w642 -> [_ w705]
          frame False {
          }
          frame True {
            n286 = call "Create RIO Data Files.vi"("Serial Numbers"=w706, "Base Filepath"=w705, "File Index In"=w708, "Anomaly Filepath In"=w710) -> ("Current Filepath"=w711:path, "File Index Out"=w707:i32, "Anomaly Filepath Out"=w709:path)  [unwired: 5 in]
          }
        }
        n287 = Open/Create/Replace File(file path (use dialog)=w648, operation (0:open)=T3."open") -> (refnum out=w675:refnum<file>, error out=w674:errorcluster)  [unwired: 4 in, 1 out]
        n288 = Select(t=w639, s=w640, f=w638) -> (s? t:f=w637:i32)
        n289 = Set File Position(refnum=w675, from (0:start)=enum16{"start", "end", "current"}."end", error in=w674) -> (refnum out=w672:refnum<file>, error out=w671:errorcluster)  [unwired: 1 in]
        n290 = Write to Text File(file (use dialog)=w672, text=w659, error in=w671) -> (refnum out=w678:refnum<file>, error out=w679:errorcluster)  [unwired: 1 in, 1 out]
        n291 = call "Handle Anomaly Log.vi"("Data"=w650, "Anomalies"=w632, "Enable"=w647, "RowCount In"=w641, "Anomaly Log Path"=w649, "Current Data Path"=w648) -> ()  [unwired: 10 in]
        n292 = Close File(refnum=w678, error in=w679) -> (path=w653:path, error out=w677:errorcluster)
        n293 = call <vilib>:"Clear Errors.vi"("error in (no error)"=w677) -> ()  [unwired: 6 in, 1 out]
        n294 = Bundle By Name(cluster=w665, "Day"=w658, "PtsTaken"=w637, "Anomaly Path"=w649, "FileIndex"=w652, "Stored Filepath"=w653) -> (w664:T2)
      }
      frame "Empty FIFO" {
        n295 = Unbundle By Name(w743) -> ("FPGA Ref"=w741:T1)
        n296 = xnode "Invoke Method"("FPGA VI Reference In"=w741, "Number of Elements"=u32 0) -> ("FPGA VI Reference Out"=w740:T1, "error out"=w739:errorcluster, "Elements Remaining"=w737:u32)  [unwired: 2 in, 1 out]
        n297 = xnode "Invoke Method"("FPGA VI Reference In"=w740, "error in"=w739, "Number of Elements"=w737) -> ()  [unwired: 1 in, 4 out]
      }
      frame "Realign FIFO" {
        n298 = Unbundle By Name(w748) -> ("FPGA Ref"=w751:T1)
        n299 = while {
          shift-right: [w759] -> w749
          shift-left: w751 -> [w760]
          stop <- w752 stop-if-true
          n300 = xnode "Invoke Method"("FPGA VI Reference In"=w760, "Number of Elements"=u32 1) -> ("FPGA VI Reference Out"=w759:T1, "Data"=w757:fxp<+/-,18,11>[])  [unwired: 2 in, 2 out]
          n301 = Index Array(array=w757, index=0) -> (element=w755:fxp<+/-,18,11>)
          n302 = In Range and Coerce(upper limit=fxp<+/-,18,5> -14.0, x=w755, lower limit=fxp<+/-,18,5> -15.0) -> (In Range?=w752:bool)  [unwired: 1 out]
        }
        n303 = Insert Into Array(array=w745, index=0, new element="Hr Record" ("new element/subarray")) -> (w744:string[])
        n304 = xnode "Invoke Method"("FPGA VI Reference In"=w749, "Number of Elements"=u32 13) -> ()  [unwired: 2 in, 4 out]
      }
      frame "Transfer Files" {
        # "Not transferring the current data or anomaly file in case they are still to be written to"
        n305 = Unbundle By Name(w765) -> ("Stored Filepath"=w764:path, "Anomaly Path"=w763:path)
        n306 = Build Array(w764, w763) -> (w761:path[])
        n307 = flat-sequence {
          tunnel: [w770] -> w762
          tunnel: w761 -> [w770]
          tunnel: w762 -> [w774]
          frame #0 {
            n308 = call "LS Data Global.vi"("Recording In"=FALSE, "Mode"=enum16{"Read", "Engine Writes", "Main Writes"}."Engine Writes", "Transferring In"=TRUE) -> ()  [unwired: 9 in, 4 out]
          }
          frame #1 {
            n309 = call "WebDAV mass transfer.vi"("Prevented Files"=w774) -> ()  [unwired: 11 in]
          }
        }
        n310 = Insert Into Array(array=w769, index=0, new element="Wait 2" ("new element/subarray")) -> (w768:string[])
      }
      frame "End Hr Record" {
        n311 = Insert Into Array(array=w778, index=0, new element="Wait" ("new element/subarray")) -> (w777:string[])
      }
      frame "Profile Record" {
        n312 = disable-structure shown="Enabled" {
          disable-tunnel: w784 -> [w810 w904]
          disable-tunnel: [w809 w904] -> w783
          disable-tunnel: w782 -> [w808 _]
          disable-tunnel: w781 -> [w791 w903]
          disable-tunnel: [w790 w903] -> w780
          frame Disabled {
            n313 = Unbundle By Name(w810) -> ("FPGA Ref"=w802:T1, "Time"=w796:dbl)
            n314 = Unbundle By Name(w808) -> ("Running?"=w793:bool, "Profile Record"=w792:bool, "RecordDuration"=w805:i32, "RecordFreq"=w806:i32, "Data Filepath"=w807:path, "RecordInterval"=w794:i32)
            n315 = Get Date/Time In Seconds() -> (seconds since 1Jan1904=w804:timestamp)
            n316 = To Double Precision Float(number=w804) -> (double precision float=w797:dbl)
            n317 = Subtract(x=w797, y=w796) -> (x-y=w801:dbl)
            n318 = Subtract(x=w794, y=w801) -> (x-y=w795:dbl)
            n319 = Empty String/Path?(string/path=w807) -> (empty?=w799:bool)
            n320 = And(x=w793, y=w792) -> (x .and. y?=w788:bool)
            n321 = Less Or Equal To 0?(x=w795) -> (x <= 0?=w800:bool)
            n322 = Compound Arithmetic op=AND(invert w799, w800) -> (w798:bool)
            n323 = Select(t="Profile Record", s=w788, f="Wait") -> (s? t:f=w785:string)
            n324 = case shown="True" w798 {
              tunnel: w806 -> [_ w841]
              tunnel: w805 -> [_ w847]
              tunnel: w802 -> [_ w844]
              tunnel: w797 -> [_ w843]
              tunnel: [w819 w843] -> w803
              tunnel: w796 -> [w819 _]
              tunnel: w795 -> [w813 _]
              tunnel: w807 -> [_ w820]
              frame False {
                w818 = u32 500 ("milliseconds to wait")
                n325 = Multiply(x=1000.0 ("y"), y=w813) -> (x*y=w815:dbl)
                n326 = To Unsigned Long Integer(number=w815) -> (unsigned 32bit integer=w812:u32)
                n327 = Less?(x=w818, y=w812) -> (x < y?=w816:bool)
                n328 = Increment(x=w812) -> (x+1=w811:u32)
                n329 = Select(t=w818, s=w816, f=w811) -> (s? t:f=w817:u32)
                n330 = Wait (ms)(milliseconds to wait=w817) -> ()  [unwired: 1 out]
              }
              frame True {
                n331 = Divide(x=1000, y=w841) -> (x/y=w846:dbl)
                n332 = Multiply(x=w847, y=w841) -> (x*y=w834:i32)
                n333 = Round Toward -Infinity(1:w846) -> (0:w848:dbl)
                n334 = Subtract(x=w846, y=w848) -> (x-y=w840:dbl)
                n335 = To Unsigned Long Integer(number=w846) -> (unsigned 32bit integer=w845:u32)
                n336 = flat-sequence {
                  tunnel: w840 -> [w851]
                  tunnel: w844 -> [w852]
                  tunnel: w845 -> [w853]
                  tunnel: w834 -> [w854]
                  tunnel: [w854] -> w839
                  tunnel: [w853] -> w838
                  tunnel: [w852] -> w837
                  tunnel: [w851] -> w836
                  tunnel: [w850] -> w829
                  tunnel: [w849] -> w821
                  tunnel: w820 -> [w849]
                  tunnel: w839 -> [w857]
                  tunnel: w838 -> [w861]
                  tunnel: w837 -> [w860]
                  tunnel: w836 -> [w855]
                  tunnel: [w859] -> w835
                  tunnel: [w858] -> w830
                  tunnel: w829 -> [w858]
                  tunnel: [w857] -> w827
                  tunnel: [w856] -> w822
                  tunnel: w821 -> [w856]
                  tunnel: w835 -> [w878]
                  tunnel: [w878] -> w833
                  tunnel: [w877] -> w832
                  tunnel: [w876] -> w831
                  tunnel: w830 -> [w876]
                  tunnel: [w875] -> w828
                  tunnel: w827 -> [w875]
                  tunnel: [w874] -> w823
                  tunnel: w822 -> [w874]
                  tunnel: w833 -> [w894]
                  tunnel: w832 -> [w888]
                  tunnel: w831 -> [w887]
                  tunnel: w828 -> [w886]
                  tunnel: [w894] -> w826
                  tunnel: [w884] -> w825
                  tunnel: [w881] -> w824
                  tunnel: w823 -> [w881]
                  tunnel: w824 -> [w900]
                  tunnel: w825 -> [w901]
                  tunnel: w826 -> [w902]
                  frame #0 {
                    n337 = Get Date/Time In Seconds() -> (seconds since 1Jan1904=w850:timestamp)
                  }
                  frame #1 {
                    n338 = for {
                      N: w857 -> [_]
                      tunnel: w861 -> [w873]
                      shift-right: [w870] -> _
                      shift-left: w855 -> [w871]
                      tunnel: w855 -> [w869]
                      tunnel: w860 -> [w868]
                      tunnel: [w866] -> w859 mode=indexing
                      n339 = xnode "Read/Write Control"("FPGA VI Reference In"=w868) -> ("Analog Inputs"=w867:fxp<+/-,28,17>[])  [unwired: 1 in, 2 out]
                      n340 = Greater Or Equal?(x=w871, y=1.0) -> (x >= y?=w864:bool)
                      n341 = Boolean To (0,1)(Boolean=w864) -> (0, 1=w863:i16)
                      n342 = Add(x=w873, y=w863) -> (x+y=w872:u32)
                      n343 = Subtract(x=w871, y=w863) -> (x-y=w862:dbl)
                      n344 = Add(x=w862, y=w869) -> (x+y=w870:dbl)
                      n345 = Wait (ms)(milliseconds to wait=w872) -> ()  [unwired: 1 out]
                      n346 = To Double Precision Float(number=w867) -> (double precision float=w866:dbl[])
                    }
                  }
                  frame #2 {
                    n347 = Get Date/Time In Seconds() -> (seconds since 1Jan1904=w877:timestamp)
                  }
                  frame #3 {
                    w883 = 86400.0 ("y")
                    n348 = To Double Precision Float(number=w888) -> (double precision float=w882:dbl)
                    n349 = To Double Precision Float(number=w887) -> (double precision float=w879:dbl)
                    n350 = Decrement(x=w886) -> (x-1=w885:i32)
                    n351 = Subtract(x=w882, y=w879) -> (x-y=w880:dbl)
                    n352 = Divide(x=w880, y=w885) -> (x/y=w889:dbl)
                    n353 = Divide(x=w889, y=w883) -> (x/y=w893:dbl)
                    n354 = Divide(x=w879, y=w883) -> (x/y=w890:dbl)
                    n355 = Add(x=w890, y=1462.0) -> (x+y=w892:dbl)
                    n356 = for {
                      N: w886 -> [_]
                      shift-right: [w895] -> _
                      shift-left: w892 -> [w896]
                      tunnel: w893 -> [w897]
                      tunnel: [w896] -> w884 mode=indexing
                      n357 = Add(x=w897, y=w896) -> (x+y=w895:dbl)
                    }
                  }
                  frame #4 {
                    n358 = call "Format Data to Save.vi"("Sections"="Sections", "FilePath"=w900, "LoopBeginWait(ms)"="LoopWait(ms)", "Time"=w901, "Data"=w902) -> ()  [unwired: 7 in]
                  }
                }
              }
            }
            n359 = Insert Into Array(array=w791, index=0, new element=w785) -> (w790:string[])
            n360 = Bundle By Name(cluster=w810, "Time"=w803) -> (w809:T2)
          }
          frame Enabled {
          }
        }
      }
    }
  }
